vi "Compute Count.vi"(8 "error in (no error)":errorcluster, 10 "Test Result":T1, 11 "Test Suite in":refnum<class "Test Suite.lvclass">) -> (0 "error out":errorcluster, 2 "Count":i32, 3 "Test Suite out":refnum<class "Test Suite.lvclass">)   [LabVIEW 2013, in "JUnit XML.lvlib" / "Test Suite.lvclass"]
uses:
  Test Suite.lvclass
  Test Case/Test Result.ctl
  Test Suite.lvclass/Test Suite.ctl
  Test Case/Test Case.lvclass/Test Case.ctl
  Test Case/Read Test Result.vi
  Test Case/Test Case.lvclass
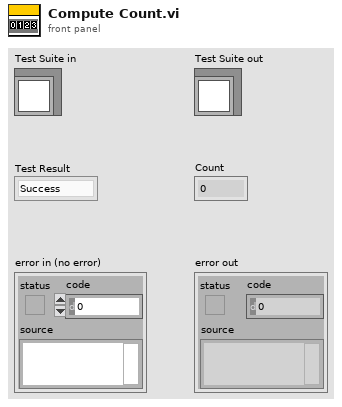
[diagram p1: front panel]
types:
  T1 = typedef "JUnit XML.lvlib/Test Case.lvclass/Test Result.ctl" = enum16{"Success", "Failure", "Error", "Skipped"}
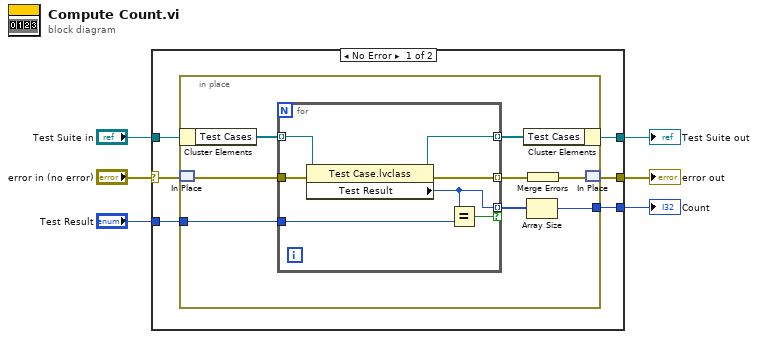
[diagram p0: block diagram]
diagram:
  n1 = case shown="No Error" "error in (no error)" {
    selector: "error in (no error)" -> [w8 w29]
    tunnel: [w7 w29] -> w5
    tunnel: [w11 w28] -> w3
    tunnel: "Test Suite in" -> [w12 w28]
    tunnel: "Test Result" -> [w10 _]
    tunnel: [w9 _] -> w1
    frame No Error {
      n2 = in-place {
        in-place-border: w10 -> [w15]
        in-place-border: [w13] -> w9
        n3 = in-place-cluster #1(w12) -> ("Test Cases"=w20:refnum<class "Test Case.lvclass">[])
        n4 = in-place-match #2(w8) -> (w18:errorcluster)
        n5 = for {
          tunnel: w20 -> [w27] mode=indexing
          tunnel: [w26] -> w19 mode=indexing
          tunnel: w18 -> [w25]
          tunnel: [w24] -> w17 mode=indexing
          tunnel: w15 -> [w23]
          tunnel: [w22] -> w14 mode=indexing if=w21
          n6 = property class="Test Case.lvclass"(reference=w27, error in=w25) -> (reference out=w26:refnum<class "Test Case.lvclass">, error out=w24:errorcluster, "Test Result"=w22:T1)
          n7 = Equal?(x=w22, y=w23) -> (x = y?=w21:bool)
        }
        n8 = in-place-cluster #1("Test Cases"=w19) -> (w11:refnum<class "Test Suite.lvclass">)
        n9 = Array Size(array=w14) -> (size(s)=w13:i32)
        n10 = Merge Errors(w17) -> (w16:errorcluster)
        n11 = in-place-match #2(w16) -> (w7:errorcluster)
      }
    }
    frame Error {
    }
  }
  "error out" <- w5
  "Test Suite out" <- w3
  "Count" <- w1
